vi "Export Data to Excel Or ClipBoard.vi"(8 "error in (no error)":errorcluster caption="错误输入（无错误）", 10 "选择区域输入":T1, 11 "Table Ref In":refnum<vi>) -> (0 "error out":errorcluster caption="错误输出", 3 "Table Ref Out":refnum<vi>)   [LabVIEW 2012, in "Table Tool.lvlib"]
uses:
  Table Tool.lvlib
  Selection Area.ctl
  <vilib>/Utility/miscctls.llb/LVRowAndColumnTypeDef.ctl
  GetOrSet.ctl
panel:
  in  "目标":enum16{"剪切板|", "Excel"}(ring)
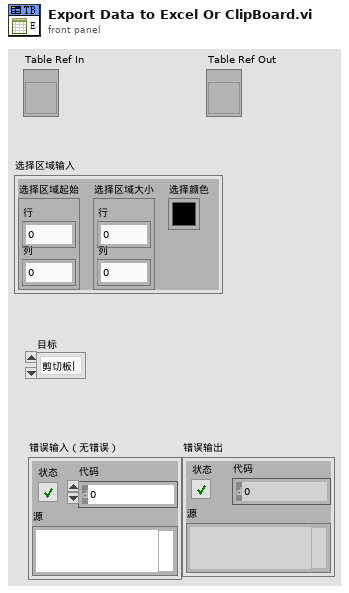
[diagram p1: front panel]
types:
  T1 = typedef "Table Tool.lvlib/Selection Area.ctl" = cluster{"选择区域起始":T2, "选择区域大小":T2, "选择颜色":u32}
  T2 = typedef "LVRowAndColumnTypeDef.ctl" = cluster{"Row":i32, "Column":i32}
  T3 = typedef "Table Tool.lvlib/GetOrSet.ctl" = enum16{"Get", "Set"}
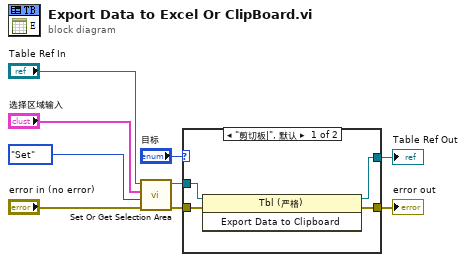
[diagram p0: block diagram]
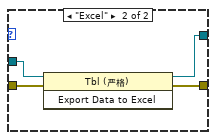
[diagram p2: hidden frame]
diagram:
  n1 = call "Set Or Get Selection Area.vi"("error in (no error)"="error in (no error)", "Mode"=GetOrSet."Set", "选择区域输入"="选择区域输入", "Table Ref In"="Table Ref In") -> ("error out"=w5:errorcluster, "Table Ref Out"=w4:refnum<vi>)  [unwired: 5 in, 1 out]
  n2 = case shown="\"剪切板|\", 默认" "目标" {
    tunnel: w5 -> [w12 w17]
    tunnel: w4 -> [w13 w16]
    tunnel: [w10 w15] -> w3
    tunnel: [w11 w14] -> w2
    frame "剪切板|", Default {
      n3 = invoke class="Tbl (严格)" method="Export Data to Clipboard"(reference=w13, error in=w12) -> (reference out=w10:refnum<vi>, error out=w11:errorcluster)  [unwired: 1 in, 1 out]
    }
    frame "Excel" {
      n4 = invoke class="Tbl (严格)" method="Export Data to Excel"(reference=w16, error in=w17) -> (reference out=w15:refnum<vi>, error out=w14:errorcluster)  [unwired: 1 in, 1 out]
    }
  }
  "Table Ref Out" <- w3
  "error out" <- w2
